vi "YZGrid.vi"() -> ()   [LabVIEW 2013]
uses:
  <vilib>/Math Plots/3D Math Plots/3D Scatter/3D Scatter XCtrl/3D Scatter.xctl
  <vilib>/gmath/interp.llb/Create Mesh Grid (2D) (x,y arrays).vi
  <vilib>/Math Plots/3D Math Plots/3D Scatter/3D Scatter Datatype/Public/Plot Helper (Matrices).vi
  <vilib>/gmath/NI_Gmath.lvlib
  <vilib>/Math Plots/3D Math Plots/3D Scatter/3D Scatter Datatype/3D Scatter Datatype.lvclass
panel:
  out "3D Scatter":refnum<class "3D Plot Datatype.lvclass">[](xcontrol)
  in  "Growth Law z":string(combo)="Linear"
  in  "h = Initial Height z":dbl
  in  "r = Height Ratio z":dbl
  in  "n = Layer Number z":i32
  in  "n = Layer Number y":i32
  in  "r = Height Ratio y":dbl
  in  "h = Initial Height y":dbl
  in  "Growth Law y":string(combo)="Linear"
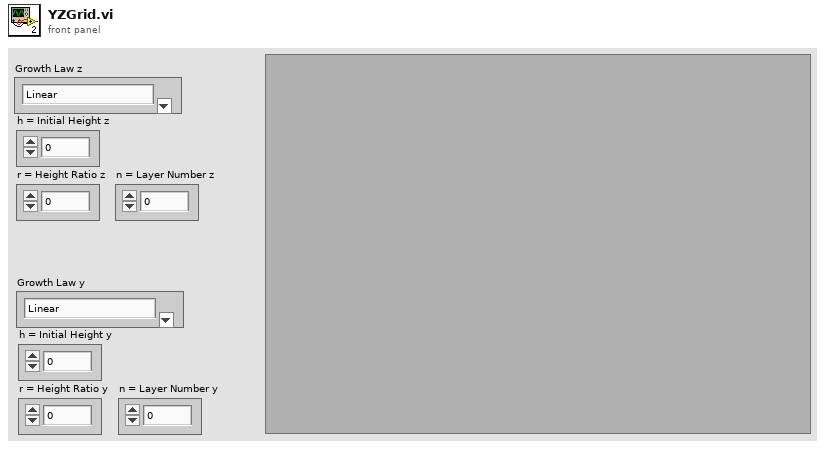
[diagram p1: front panel]
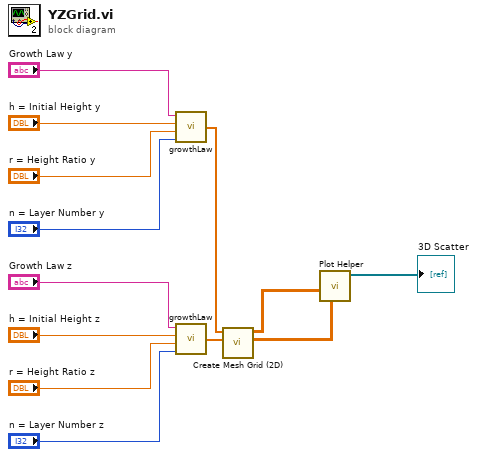
[diagram p0: block diagram]
diagram:
  n1 = call "growthLaw.vi"("n = Layer Number"="n = Layer Number y", "r = Height Ratio"="r = Height Ratio y", "h = Initial Height"="h = Initial Height y", "Growth Law"="Growth Law y") -> ("Coordinates"=w5:dbl[])
  n2 = call "growthLaw.vi"("n = Layer Number"="n = Layer Number z", "r = Height Ratio"="r = Height Ratio z", "h = Initial Height"="h = Initial Height z", "Growth Law"="Growth Law z") -> ("Coordinates"=w4:dbl[])
  n3 = call-poly <vilib>:"Create Mesh Grid (2D).vi"("y domain"=w4, "x domain"=w5) -> ("Y"=w1:dbl[][], "X"=w2:dbl[][])  [unwired: 7 in, 1 out]
  n4 = call-poly <vilib>:"Plot Helper.vi"("z matrix"=w1, "y matrix"=w2) -> ("3D Plot lvclass Array out"=→"3D Scatter":refnum<class "3D Plot Datatype.lvclass">[])  [unwired: 4 in, 5 out]
